vi "Apply Default.vi"(11 "ID in":refnum<class "ID.lvclass">) -> (3 "ID out":refnum<class "ID.lvclass">)   [LabVIEW 2020, in "Conditu2.lvlib" / "Columns.lvlib" / "ID.lvclass"]
uses:
  ID.lvclass
  Type/Type.lvclass
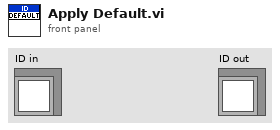
[diagram p1: front panel]
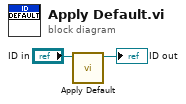
[diagram p0: block diagram]
diagram:
  n1 = call-parent "Apply Default.vi"("Type in"="ID in") -> ("Type out"=→"ID out":refnum<class "ID.lvclass">)  [unwired: 10 in]
